vi "PostCopyScripting.vi"(10 "MetaDataObj":refnum<class "MetaDataObj.lvclass">, 11 "User Project":refnum<vi>) -> ()   [LabVIEW 2013, in "FixedChannelTBModuleDecideFeatures.lvclass"]
uses:
  FixedChannelTBModuleDecideFeatures.lvclass
  <resource>/dialog/NewProjectWizard/MetaDataObj/MetaDataObj.lvclass
  FixedChannelTBModuleDecideFeatures.lvclass/FixedChannelTBModuleDecideFeatures.ctl
  Read component name.vi
  Read Channel Specification.vi
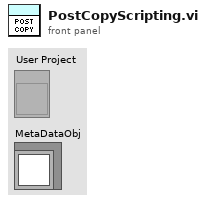
[diagram p1: front panel]
types:
  T1 = typedef "channel configuration.ctl" = cluster{"Name":string, "channel classification":T2, "data type":T3}
  T2 = typedef "TBM channel.lvclass/channel classification.ctl" = enum16{"input data", "output data", "processing parameter", "processing result"}
  T3 = typedef "tag bus.lvlib/tag descriptor.lvclass/Data Type.ctl" = enum16{"Double", "Single", "I64", "I32", "I16", "I8", "U64", "U32", "U16", "U8", "Boolean", "String", "Array of Double", "Array of Single", "Array of I64", "Array of I32", "Array of I16", "Array of I8", "Array of U64", "Array of U32", "Array of U16", "Array of U8", "Array of Boolean", "Array of String"}
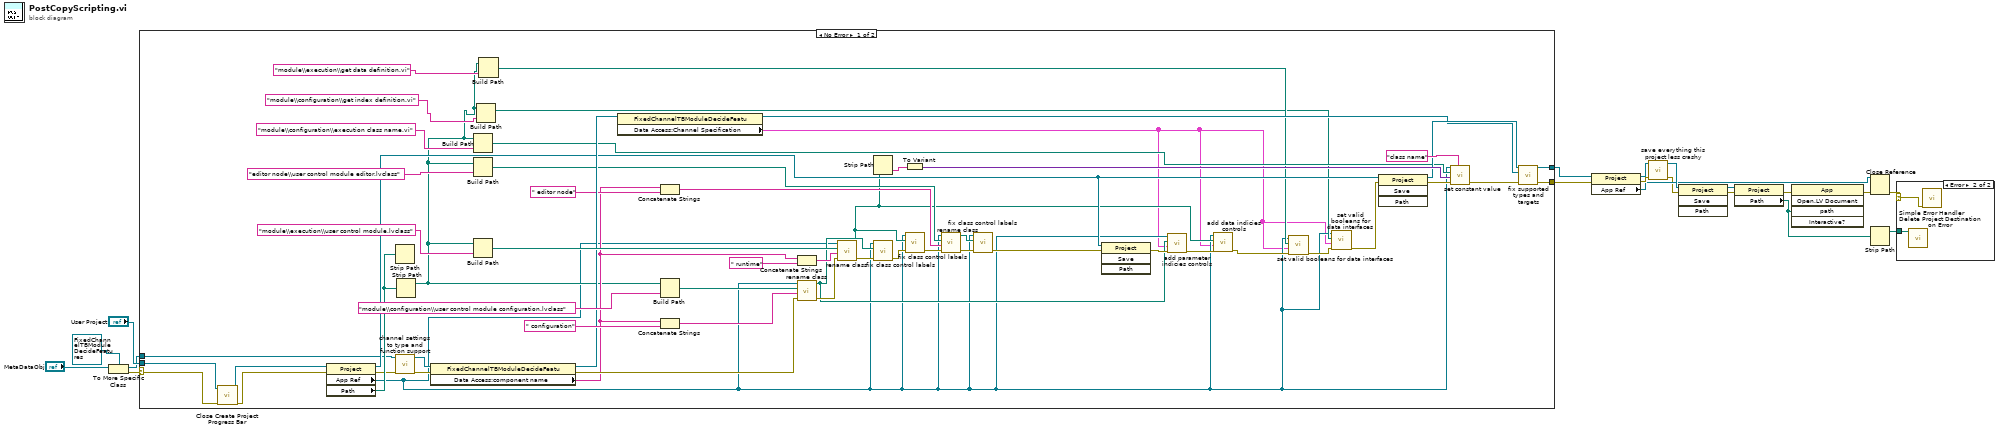
[diagram p0: block diagram]
diagram:
  n1 = To More Specific Class(target class=refnum<class "FixedChannelTBModuleDecideFeatures.lvclass"> refnum ("DecideProjectFeatures.lvclass"), reference="MetaDataObj") -> (specific class reference=w10:refnum<class "FixedChannelTBModuleDecideFeatures.lvclass">, error out=w17:errorcluster)  [unwired: 1 in]
  n2 = case shown="No Error" w17 {
    selector: w17 -> [w32 w77]
    tunnel: [w56 w78] -> w1
    tunnel: "User Project" -> [w33 w78]
    tunnel: [w57 w77] -> w2
    tunnel: w10 -> [w41 _]
    frame No Error {
      n3 = call <resource>:"Close Create Project Progress Bar.vi"("error in (no error)"=w32, "Project"=w33) -> ("error out"=w31:errorcluster, "dup Project"=w30:refnum<vi>)  [unwired: 8 in]
      n4 = property class="Project"(reference=w30, error in=w31) -> (reference out=w46:refnum<vi>, error out=w40:errorcluster, "App Ref"=w21:refnum<vi>, "Path"=w45:path)
      n5 = Strip Path(path=w45) -> ()  [unwired: 2 out]
      n6 = call "channel settings to type and function support.vi"("error in"=w40, "FixedChannelTBModuleDecideFeatures in"=w41) -> ("error out"=w43:errorcluster, "FixedChannelTBModuleDecideFeatures out"=w42:refnum<class "FixedChannelTBModuleDecideFeatures.lvclass">)  [unwired: 8 in]
      n7 = Strip Path(path=w45) -> (stripped path=w27:path)  [unwired: 1 out]
      n8 = property class="FixedChannelTBModuleDecideFeatu"(reference=w42, error in=w43) -> (reference out=w72:refnum<class "FixedChannelTBModuleDecideFeatures.lvclass">, error out=w44:errorcluster, "Data Access:component name"=w35:string)
      n9 = Build Path(base path=w27, name or relative path="module\\configuration\\execution class name.vi") -> (appended path=w39:path)
      n10 = Build Path(base path=w27, name or relative path="editor node\\user control module editor.lvclass") -> (appended path=w63:path)
      n11 = Build Path(base path=w27, name or relative path="module\\execution\\user control module.lvclass") -> (appended path=w74:path)
      n12 = Build Path(base path=w27, name or relative path="module\\configuration\\get index definition.vi") -> (appended path=w22:path)
      n13 = Build Path(base path=w27, name or relative path="module\\execution\\get data definition.vi") -> (appended path=w25:path)
      n14 = property class="FixedChannelTBModuleDecideFeatu"(reference=w72) -> (reference out=w48:refnum<class "FixedChannelTBModuleDecideFeatures.lvclass">, "Data Access:Channel Specification"=w20:T1[])  [unwired: 1 in, 1 out]
      n15 = Concatenate Strings(w35, " editor node" ("string")) -> (w58:string)
      n16 = Build Path(base path=w27, name or relative path="module\\configuration\\user control module configuration.lvclass") -> (appended path=w49:path)
      n17 = Concatenate Strings(w35, " configuration" ("string")) -> (w54:string)
      n18 = Concatenate Strings(w35, " runtime" ("string")) -> (w51:string)
      n19 = call "rename class.vi"("error in"=w44, "new name"=w54, "class path"=w49, "Application in"=w21) -> ("error out"=w50:errorcluster, "New Library Path"=w38:path)  [unwired: 6 in]
      n20 = call "rename class.vi"("error in"=w50, "new name"=w51, "class path"=w74, "Application in"=w21) -> ("error out"=w66:errorcluster, "New Library Path"=w36:path)  [unwired: 6 in]
      n21 = Strip Path(path=w36) -> (name=w53:string)  [unwired: 1 out]
      n22 = call "fix class control labels.vi"("error in"=w66, "class to load"=w38, "Application in"=w21) -> ("error out"=w65:errorcluster)  [unwired: 8 in]
      n23 = To Variant(anything=w53) -> (Variant=w71:variant)
      n24 = call "fix class control labels.vi"("error in"=w65, "class to load"=w36, "Application in"=w21) -> ("error out"=w60:errorcluster)  [unwired: 8 in]
      n25 = call "rename class.vi"("error in"=w60, "new name"=w58, "class path"=w63, "Application in"=w21) -> ("error out"=w61:errorcluster, "New Library Path"=w62:path)  [unwired: 6 in]
      n26 = call "fix class control labels.vi"("error in"=w61, "class to load"=w62, "Application in"=w21) -> ("error out"=w34:errorcluster)  [unwired: 8 in]
      n27 = invoke class="Project" method="Save"(reference=w46, error in=w34) -> (error out=w47:errorcluster)  [unwired: 2 in, 3 out]
      n28 = call "add parameter indicies controls.vi"("error in"=w47, "Channels to create"=w20, "cfg class path"=w38, "Application in"=w21) -> ("error out"=w37:errorcluster)  [unwired: 7 in]
      n29 = call "add data indicies controls.vi"("error in"=w37, "Channels to create"=w20, "runtime class path"=w36, "Application in"=w21) -> ("error out"=w26:errorcluster)  [unwired: 7 in]
      n30 = call "set valid booleans for data interfaces.vi"("error in"=w26, "Channel Specification"=w20, "vi path"=w25, "Application in"=w21) -> ("error out"=w24:errorcluster)  [unwired: 7 in]
      n31 = call "set valid booleans for data interfaces.vi"("error in"=w24, "Channel Specification"=w20, "vi path"=w22, "Application in"=w21) -> ("error out"=w23:errorcluster)  [unwired: 7 in]
      n32 = invoke class="Project" method="Save"(reference=w46, error in=w23) -> (reference out=w67:refnum<vi>, error out=w68:errorcluster)  [unwired: 2 in, 2 out]
      n33 = call "set constant value.vi"("control name"="class name", "error in"=w68, "data to set"=w71, "vi path"=w39, "Application in"=w21) -> ("error out"=w55:errorcluster)  [unwired: 6 in]
      n34 = call "fix supported types and targets.vi"("error in"=w55, "DecideProjectFeatures in"=w48, "User Project in"=w67) -> ("error out"=w57:errorcluster, "User Project out"=w56:refnum<vi>)  [unwired: 7 in]
    }
    frame Error {
    }
  }
  n35 = property class="Project"(reference=w1, error in=w2) -> (reference out=w7:refnum<vi>, error out=w8:errorcluster, "App Ref"=w6:refnum<vi>)
  n36 = call "save everything this project less crashy.vi"("error in"=w8, "Project in"=w7) -> ("error out"=w3:errorcluster, "Project out"=w9:refnum<vi>)  [unwired: 8 in]
  n37 = invoke class="Project" method="Save"(reference=w9, error in=w3) -> (reference out=w13:refnum<vi>, error out=w14:errorcluster)  [unwired: 2 in, 2 out]
  n38 = property class="Project"(reference=w13, error in=w14) -> (error out=w16:errorcluster, "Path"=w11:path)  [unwired: 1 out]
  n39 = invoke class="App" method="Open.LV Document"(error in=w16, "path"=w11) -> (error out=w15:errorcluster)  [unwired: 3 in, 4 out]
  n40 = Close Reference(reference=w6, error in (no error)=w15) -> (error out=w5:errorcluster)
  n41 = Strip Path(path=w11) -> (stripped path=w4:path)  [unwired: 1 out]
  n42 = case shown="Error" w5 {
    selector: w5 -> [_ w79]
    tunnel: w4 -> [_ w80]
    frame No Error {
    }
    frame Error {
      n43 = call <resource>:"Delete Project Destination on Error.vi"("Project Destination Root"=w80) -> ()  [unwired: 11 in]
      n44 = call <vilib>:"Simple Error Handler.vi"("error in (no error)"=w79) -> ()  [unwired: 4 in, 5 out]
    }
  }
